vi "RT Main.vi"() -> ()   [LabVIEW 2021]
panel:
  out "Loop Time [ms]":u32
  in  "stop":bool
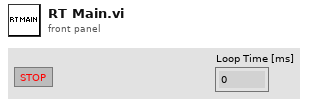
[diagram p1: front panel]
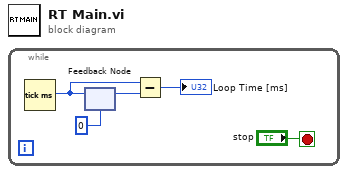
[diagram p0: block diagram]
diagram:
  n1 = while {
    stop <- "stop" stop-if-true
    n2 = Tick Count (ms)() -> (millisecond timer value=w2:u32)
    n3 = feedback-in #1(w2) -> ()
    n4 = feedback #1(u32 0 ("millisecond timer value")) -> (w3:u32)
    n5 = Subtract(x=w2, y=w3) -> (x-y=→"Loop Time [ms]":u32)
  }
